vi "GUI_HTT_CTRLv4_2013.vi"() -> ()   [LabVIEW 2020]
uses:
  Shared/GUI_Template/GUI_master/tcp_new_data_event.ctl
  Shared/GUI_Template/GUI_master/tcp new data cluster.ctl
  <vilib>/Utility/config.llb/Write Key (I32).vi
  <vilib>/Platform/browser.llb/Open URL in Default Browser (string).vi
  <vilib>/Utility/config.llb/NI_LVConfig.lvlib
panel:
  in  "Create Log":bool caption="LogTable"
  in  "Scan":T1(ring)
  out "standard output":string
  in  "LogEpilog":bool caption="LogTable"
  in  "New Google\nExpLog for new day?":bool=TRUE
  in  "LogTable":bool
  in  "PicoL2":bool caption="PicoL GUI"
  in  "1Wire B GUI":bool caption="PicoL GUI"
  out "fire::12":string="fire" caption="fire"
  in  "Wavelength.Channel0::14":enum16{"248", "355", "532", "800", "2940"}(ring)=enum."532"
  in  "Wavelength.Channel1::14":enum16{"248", "355", "532", "800", "2940"}(ring)=enum."800"
  in  "Wavelength.Channel0::13":enum16{"532", "800"}(ring)=enum."800"
  in  "EnergyRange.Channel0::14":T2(ring)=enum."400mJ"
  in  "EnergyRange.Channel1::14":T2(ring)=enum."400mJ"
  in  "EnergyRange.Channel0::13":T3(ring)=enum."200mJ"
  in  "energy.channel 1::14":dbl caption="Energy Gaia" min=0.0 max=200.0 format="%#_13g"
  out "Energy (J)":dbl
  in  "Multiplicator":dbl=15.3
  in  "GUIdevice 14":string="HTT-Energy-S-G"
  in  "Multiplicator":dbl=66.6
  in  "Multiplicator Scatter":dbl=100.0
  out "Energy Scatter (J)":dbl
  out "Energy (J)":dbl
  in  "energy.channel 0::13":dbl caption="Energy Drive" min=0.0 max=10.0 format="%#_13g"
  in  "energy.channel 0::14":dbl caption="Energy Scatter" min=0.0 max=20.0 format="%#_13g"
  in  "GUIdevice 13":string="HTT-Energy-D"
  in  "IR Pt Exp And Comp":bool caption="PicoL GUI"
  in  "Position.Axis 2::10":dbl caption="y/vert." min=-6000.0 max=6000.0
  in  "Position.Axis 3::10":dbl caption="Scatter Mode z" min=-20.0 max=20.0
  in  "Position.Axis 1::10":dbl caption="x/hor." min=-150.0 max=150.0
  in  "Position.Axis 2::11":dbl caption="Translation" min=-50.0 max=50.0
  in  "Position.Axis 3::11":dbl caption="Rotation G1" min=-360.0 max=360.0
  in  "Position.Axis 1::11":dbl caption="Rotation G2" min=-360.0 max=360.0
  in  "Ethernet Powerstrip":bool caption="Google Drive"
  in  "Position.Axis 3::4":dbl caption="z" min=-10.0 max=26.0
  in  "Position.Axis 2::6":dbl caption="Delay Stage" min=-6000.0 max=6000.0
  in  "FilterWheelB1":bool caption="PicoB GUI"
  in  "Search Log":bool caption="PicoL GUI"
  in  "Experiment \n(if, shadow, topjet)":bool caption="PicoL GUI"
  in  "RemoteDesktop":bool caption="PicoL GUI"
  in  "Experiment \n(e-profile, xrays)":bool caption="PicoL GUI"
  in  "IR TC Pointing (17s)":bool caption="PicoL GUI"
  in  "Scatter Depletion":bool caption="PicoL GUI"
  in  "Scatter IR Amps":bool caption="PicoL GUI"
  in  "Drive TC Pt":bool caption="PicoL GUI"
  in  "Gaia Profiles":bool caption="PicoL GUI"
  in  "Gaia Pointing":bool caption="PicoL GUI"
  in  "IR Exp and Comp":bool caption="PicoL GUI"
  in  "HTT Interactive":bool caption="PicoL GUI"
  in  "GUIdevice 12":string="HTT_DG645"
  in  "Delay.Ch C::12":dbl caption="Delay" min=-0.1 max=2.0 format="%#_6e"
  in  "Delay.Ch D::12":dbl caption="Width" min=-0.1 max=2.0 format="%#_6e"
  in  "Amplitude.Ch CD::12":dbl caption="DG645" min=0.5 max=5.0
  in  "Field::1":dbl caption="B-Field" min=0.0 max=10000.0
  in  "Delay.Ch 1::8":dbl caption="Delay" min=0.0 max=10.0 format="%#_6e"
  in  "Width.Ch 1::8":dbl caption="Width" min=0.0 max=1.0 format="%#_6e"
  in  "Amplitude.Ch 1::8":dbl caption="Cam Trig Amp" min=0.0 max=12.0
  in  "1Wire L GUI":bool caption="PicoL GUI"
  in  "Opt. Spectrometer":bool caption="PicoL GUI"
  in  "SingleCamGUI":bool caption="PicoL GUI"
  in  "Exp Editor":bool caption="PicoL GUI"
  in  "DB Editor":bool caption="PicoL GUI"
  in  "AddColumns":bool caption="PicoL GUI"
  in  "GEECSplot":bool caption="PicoL GUI"
  in  "LVStarter":bool caption="PicoL GUI"
  in  "MasterControl":bool caption="PicoL GUI"
  in  "MagSpecGUI":bool caption="PicoL GUI"
  in  "Google Drive":bool
  in  "Depletion Cams":bool caption="PicoL GUI"
  in  "D-L-Cams":bool caption="PicoL GUI"
  in  "Position.Axis 2::5":dbl caption="Mode Out z" min=-150.0 max=150.0
  in  "Position.Axis 1::4":dbl caption="Blade" min=-20.0 max=20.0
  in  "Amplitude.Ch 5::8":dbl caption="Trigger Amplitude (V)" min=0.0 max=12.0
  in  "Position.Axis 3::5":dbl caption="Drive Mode In z" min=-200.0 max=200.0
  in  "Position.Axis 1::5":dbl caption="Mode Out Wedge" min=-150.0 max=150.0
  out "Position.Axis3::2":dbl caption="Rotation G1" min=-180.0 max=180.0 format="%#_13g"
  out "Position.Axis2::2":dbl caption="Rotation G2" min=-180.0 max=180.0 format="%#_13g"
  in  "Position.Axis1::2":dbl caption="Translation" min=-60000.0 max=60000.0 format="%#_13g"
  in  "PicoL":bool caption="PicoL GUI"
  in  "PicoB":bool caption="PicoB GUI"
  in  "AnalogOutput.Channel 0::9":dbl caption="Pressure Ctrl (V)" min=0.0 max=10.0
  in  "Width.Ch 5::8":dbl caption="Opening time (s)" min=0.0 max=0.025 format="%#_6e"
  in  "Jet enable":bool caption="Jet Enable"
  in  "Jet trigger":bool caption="Jet Trigger"
  in  "Position.Axis 3::3":dbl caption="Jet Z" min=-25.0 max=25.0
  in  "Position.Axis 2::3":dbl caption="Jet Y" min=-25.0 max=25.0
  in  "Position.Axis 1::3":dbl caption="Jet X" min=-25.0 max=25.0
  in  "Position.Axis 3::6":dbl caption="Probe delay" min=-100.0 max=100.0
  in  "GUIdevice 11":string="HTT-ESP05"
  in  "GUIdevice 8":string="HTT-BNC"
  in  "GUIdevice 6":string="HTT-ESP04"
  in  "GUIdevice 5":string="HTT-ESP03"
  out "error IO 2":errorcluster
  out "fire::10":string
  out "tcp data event":T4
  in  "UDP error message":string
  in  "GUIdevice 7":string="HTT-Pulsar"
  in  "GUIdevice 2":string="Aerotech-HTT"
  in  "GUIdevice 10":string="HTT-ESP06"
  in  "GUIdevice 4":string="HTT-ESP02"
  in  "GUIdevice 1":string="HTT-MagTeslameter-DTM141"
  in  "GUIdevice 3":string="HTT-ESP01"
  in  "GUIdevice 9":string="HTT-HighPressureDAQ"
  in  "Delay.Ch 5::8":dbl caption="Jet timing (s)" min=0.0 max=10.0 format="%#_6e"
  in  "stop":bool
  # "Energy"
  # "CAP"
  # "HTT CONTROL CENTER"
  # "v0.5   04/01/2020"
  # "Drive"
  # "Gas Jet"
  # "GUI Collection"
  # "Compressor"
  # "Drive Cameras"
  # "Mode Imager"
  # "Probe Delay Line"
  # "Scatter Cameras"
  # "Scatter"
  # "Compressor"
  # "Electronics"
  # "BNC"
  # "Mode Imager"
  # "Experiment GUIs"
  # "Scatter Delay vs. Drive"
  # "Turning Mirror"
  # "MC Links"
  # "Docu"
  # "Log Maker"
  # "Energy"
  # "Drive"
  # "Scatter"
  # "Gaia"
  # "Adjustment GUIs"
  # "Range"
  # "Wavelength"
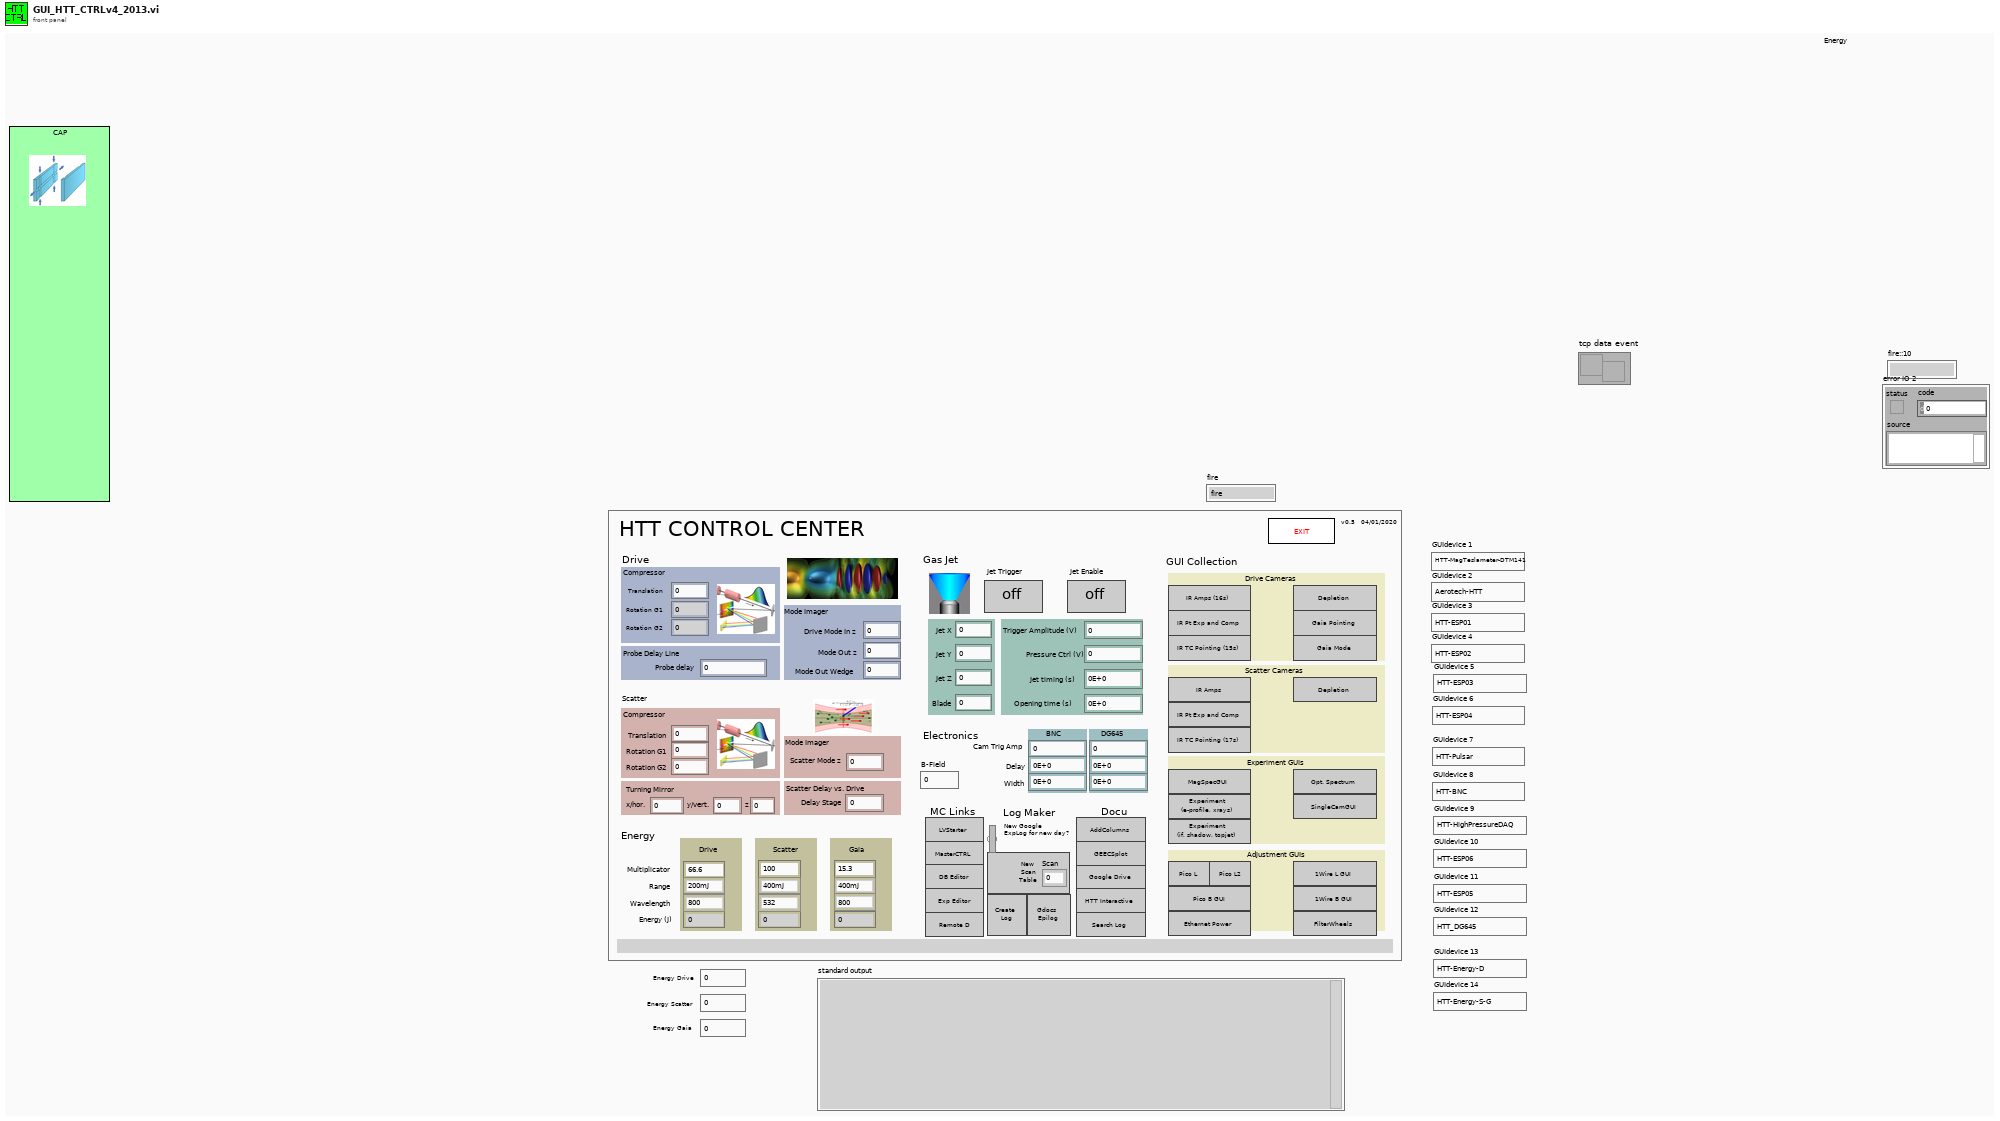
[diagram p1: front panel]
types:
  T1 = enum16{"0", "1", "2", "3", "4", "5", "6", "7", "8", "9", "10", "11", "12", "13", "14", "15", "16", "17", "18", "19", "20", "21", "22", "23", "24", "25", "26", "27", "28", "29", "30", "31", "32", "33", "34", "35", "36", "37", "38", "39", "40", "41", "42", "43", "44", "45", "46", "47", "48", "49", "50", "51", "52", "53", "54", "55", "56", "57", "58", "59", "60", "61", "62", "63", "64", "65", "66", "67", "68", "69", "70", "71", "72", "73", "74", "75", "76", "77", "78", "79", "81", "82", "83", "84", "85", "86", "87", "88", "89", "90", "91", "92", "93", "94", "95", "96", "97", "98", "99", ""}
  T2 = enum16{"4.00mJ", "40.0mJ", "400mJ", "4.00J", "20.00J"}
  T3 = enum16{"2.00mJ", "20.0mJ", "200mJ", "2.00J", "10J"}
  T4 = typedef "tcp_new_data_event.ctl" = refnum<user-event>
  T5 = typedef "tcp new data cluster.ctl" = cluster{"EventEnum":enum16{"new data", "connection status update"}, "Device name":string}
  T6 = enum32{"invalid app kind", "Development System", "Run Time System", "Student Edition", "Embedded LabVIEW", "Evaluation", "Custom"}
  T7 = enum32{"Invalid", "Standard", "Closed", "Hidden", "Minimized", "Maximized"}
  T8 = cluster{"Core":cluster{"Current VI Reference":refnum<vi>, "Close Panel on Exit?":bool}, "Heater timing offset":dbl, "Discharge timing offset":dbl, "Jet trigger":bool, "Tik1":u32, "Tik2":u32, "Fire Continues Allowed":bool, "Jet enable":bool}
  T9 = typedef "imagedata.ctl" = cluster{"image type":i32, "image depth":i32, "image":u8[], "mask":u8[], "colors":u32[], "Rectangle":cluster{"left":i16, "top":i16, "right":i16, "bottom":i16}}
  T10 = typedef "NI_LVConfig.lvlib/Config Data RefNum.ctl" = refnum<k1>
  T11 = cluster{"Current VI Reference":refnum<vi>, "Close Panel on Exit?":bool}
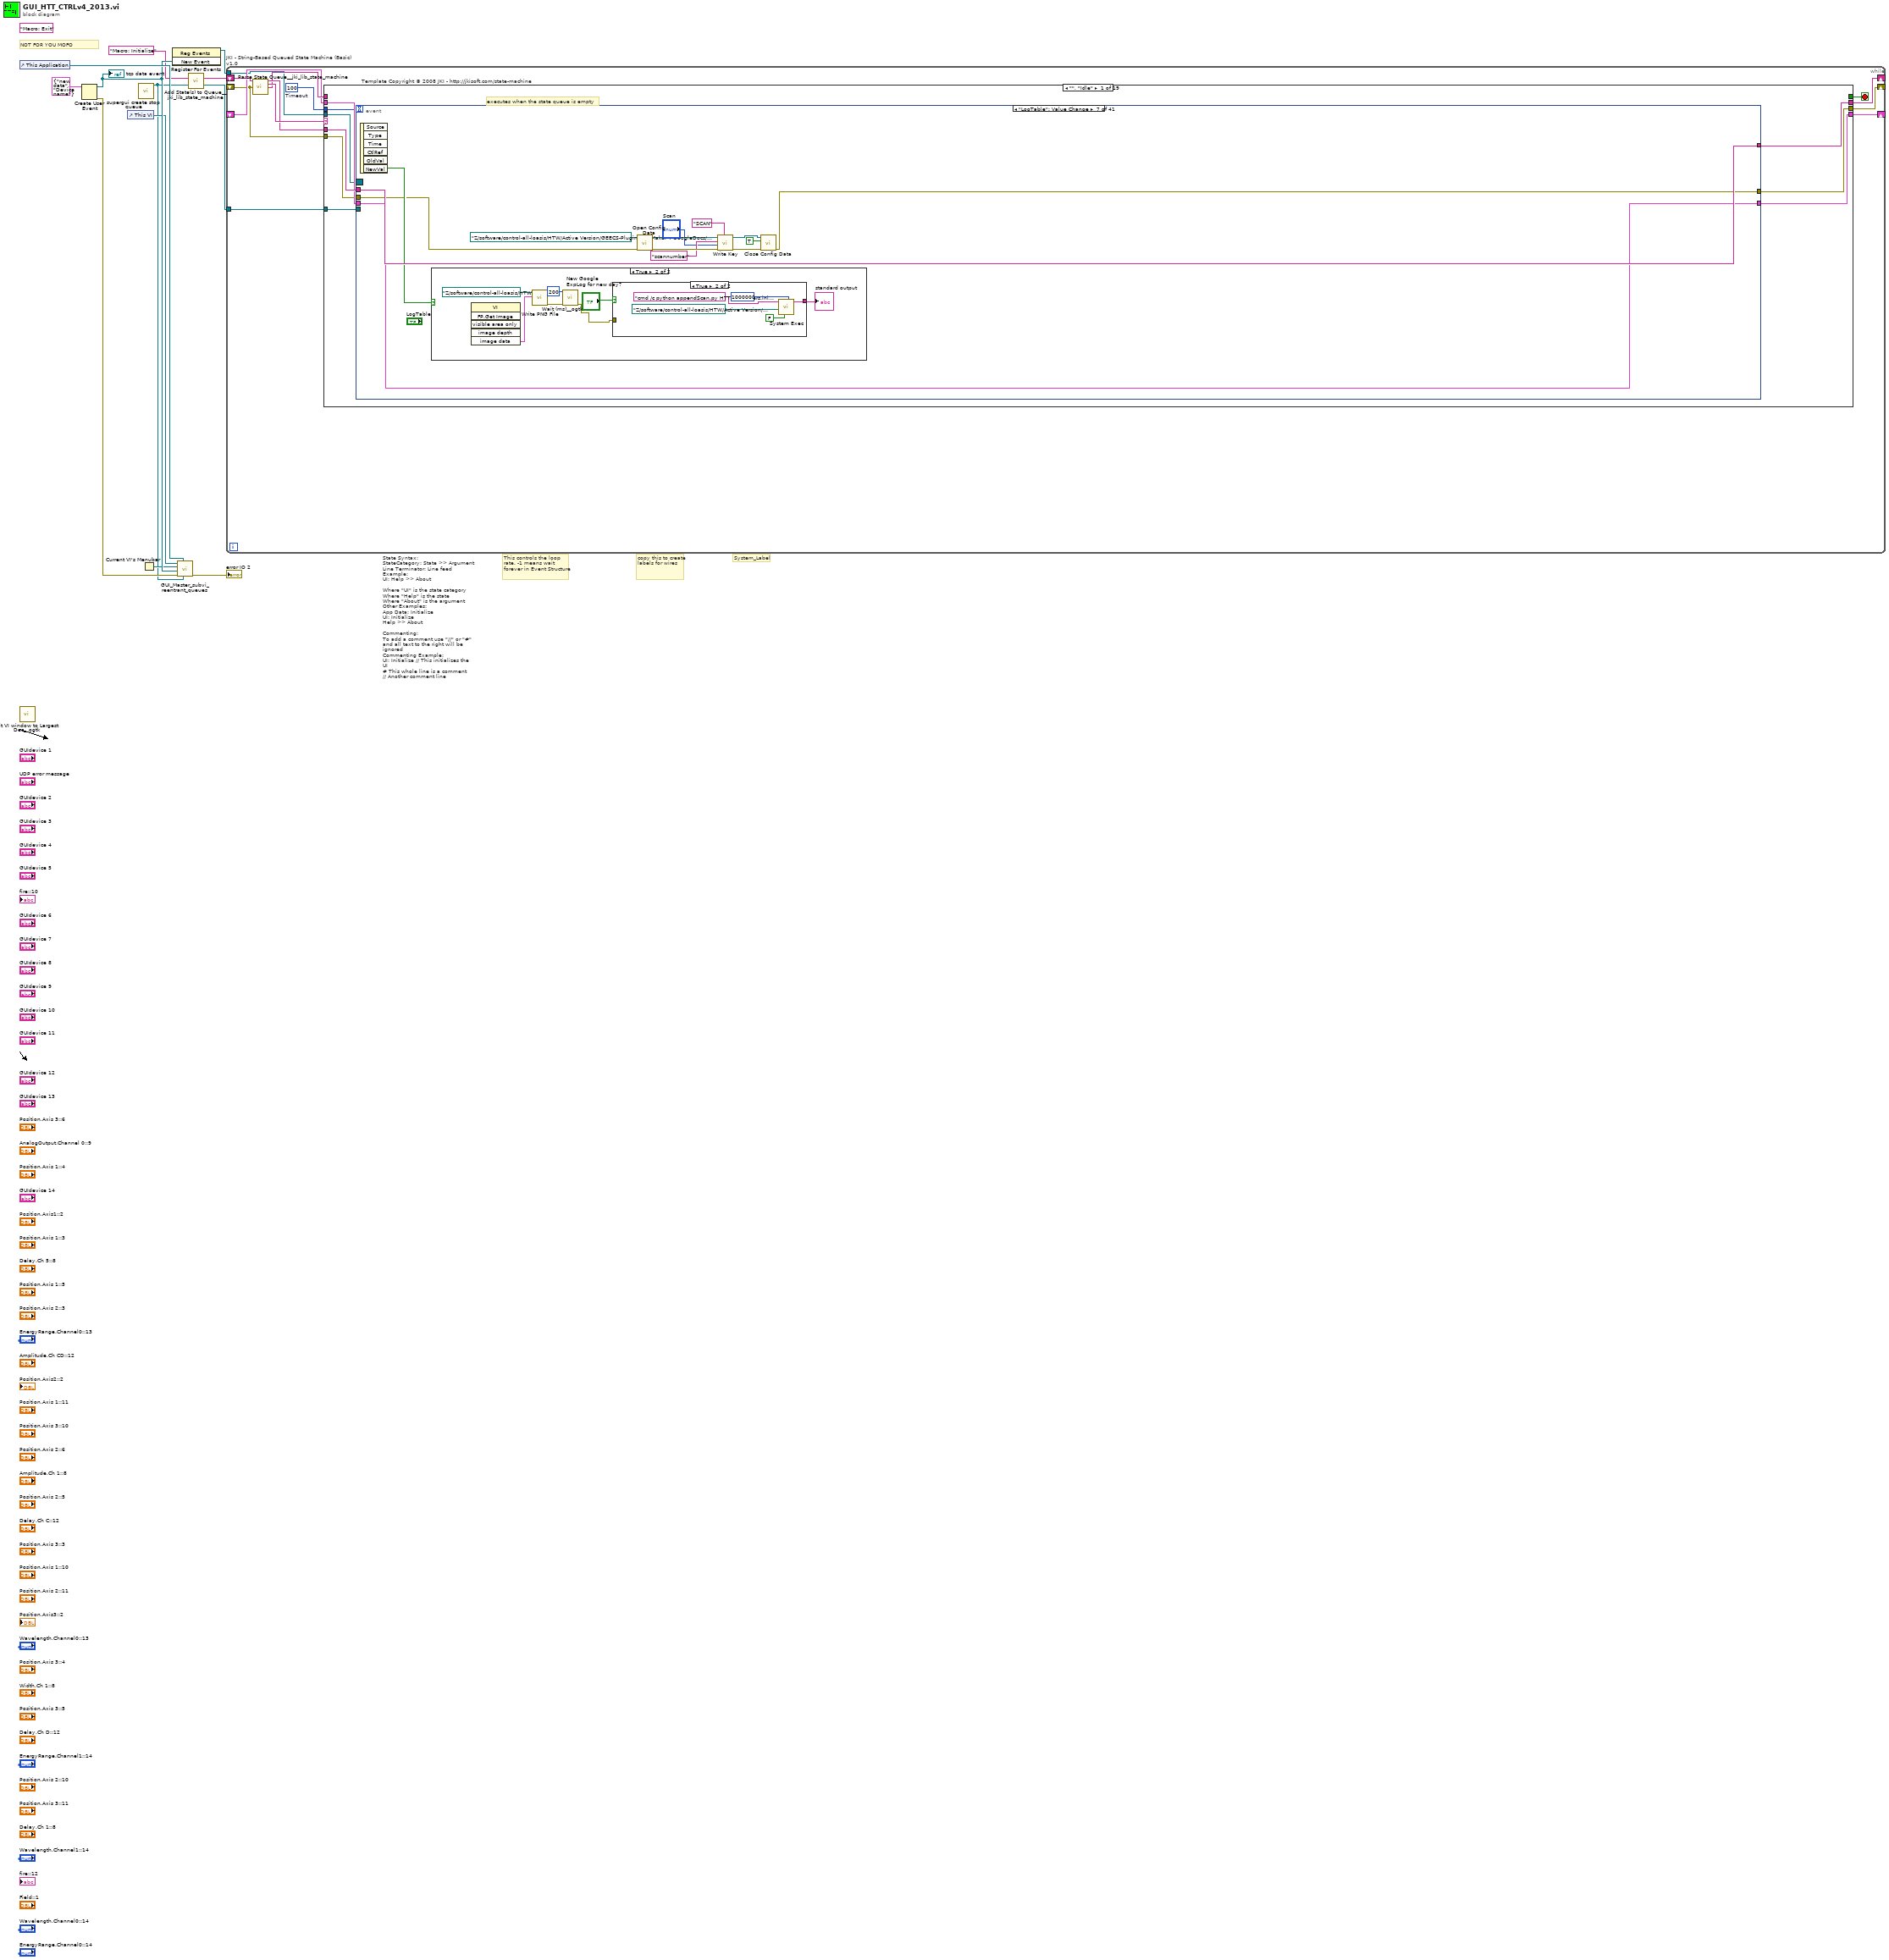
[diagram p0: block diagram]
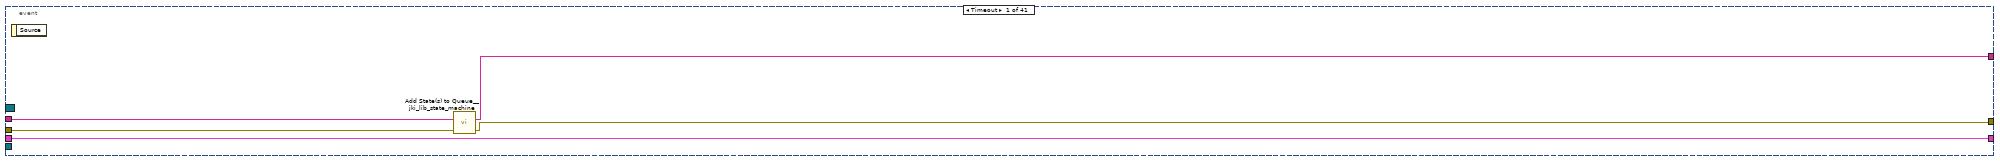
[diagram p2: hidden frame]
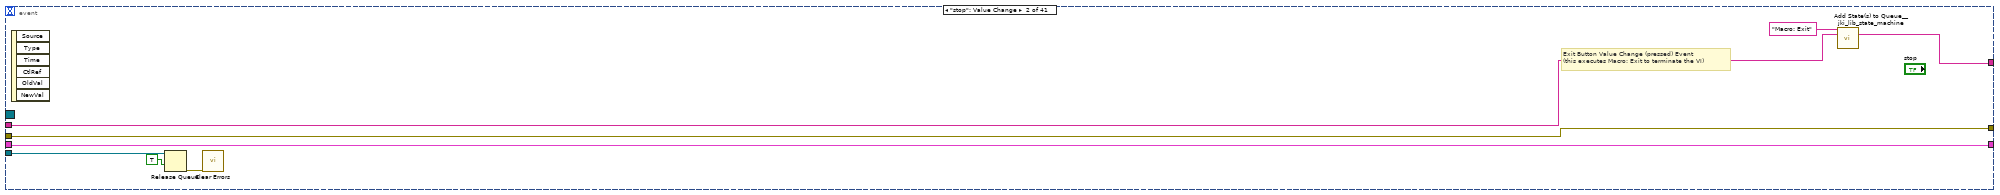
[diagram p3: hidden frame]
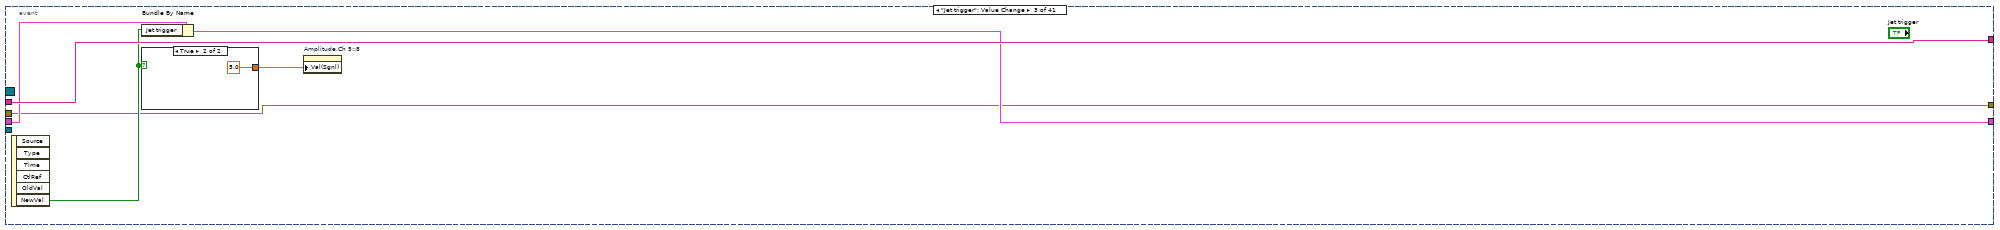
[diagram p4: hidden frame]
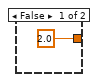
[diagram p5: hidden frame]
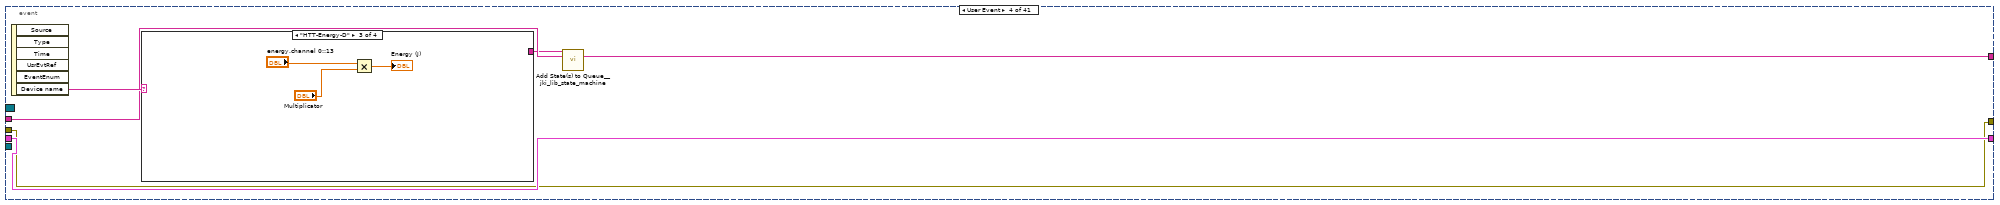
[diagram p6: hidden frame]
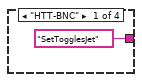
[diagram p7: hidden frame]
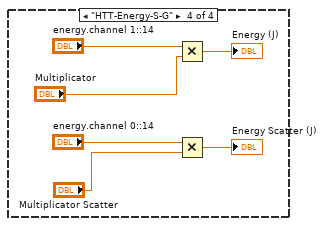
[diagram p9: hidden frame]
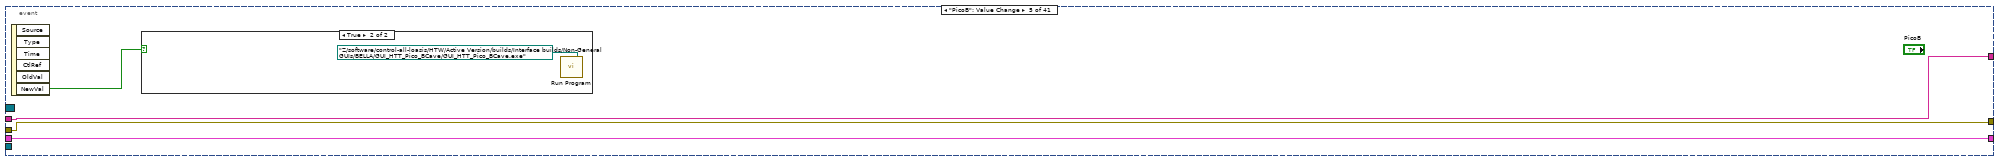
[diagram p10: hidden frame]
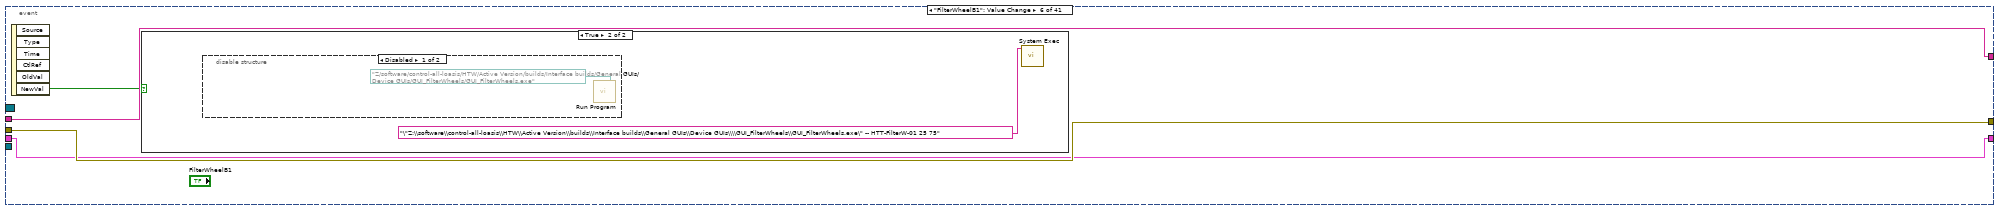
[diagram p12: hidden frame]
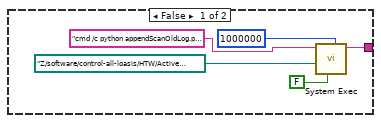
[diagram p16: hidden frame]
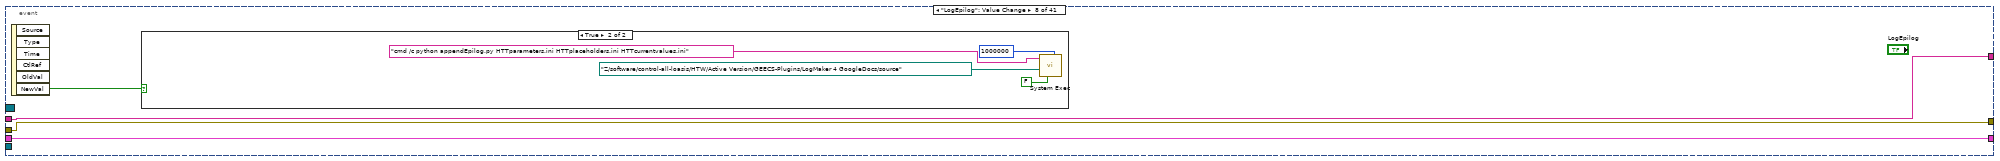
[diagram p17: hidden frame]
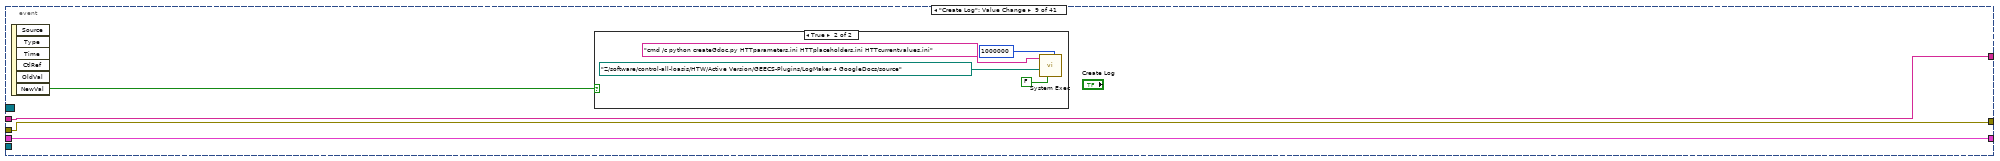
[diagram p19: hidden frame]
diagram:
  (unwired) "Macro: Exit"
  # "State Syntax:\nStateCategory: State >> Argument\nLine Terminator: Line feed\nExample:\nUI: Help >> About\n\nWhere \"UI\" is the state category\nWhere \"Help\" is the state\nWhere \"About\" is the argument\nOther Examples:\nApp Data: Initialize\nUI: Initialize\nHelp >> About\n\nCommenting:\nTo add a comment use \"//\" or \"#\" and all text to the right will be ignored\nCommenting Example:\nUI: Initialize // This initializes the UI\n# This whole line is a comment\n// Another comment line"
  # "copy this to create labels for wires"
  # "This controls the loop rate. -1 means wait forever in Event Structure"
  # "System_Label"
  # "NOT FOR YOU MOFO"
  n1 = control-ref of="This Application"() -> (w11:refnum<vi>)
  n2 = call <userlib>:"Fit VI window to Largest Dec__ogtk.vi"() -> ()  [unwired: 6 in, 2 out]
  n3 = Create User Event(user event datatype=T5 {"EventEnum"=enum."new data", "Device name"="Device name"} ("New Event")) -> (user event=w10:refnum<user-event>, error out=w9:errorcluster)  [unwired: 1 in]
  "tcp data event" <- w10
  n4 = control-ref of="This VI"() -> (w5:refnum<vi>)
  n5 = call "supergui create stop queue.vi"() -> ("STOP Queue out"=w2:refnum<queue>)  [unwired: 11 in]
  n6 = Current VI's Menubar() -> (w7:refnum<k9>)
  n7 = register-events(w10) -> (reference out=w1:refnum<event-registration>)  [unwired: 2 in, 1 out]
  n8 = call "GUI_Master_subvi_reentrant_queues.vi"("STOP Queue in"=w2, "This Application"=w11, "error in (no error)"=w9, "tcp data event"=w10, "Caller menu reference"=w7, "Caller VI ref"=w5) -> ("error out"=→"error IO 2":errorcluster)  [unwired: 5 in]
  n9 = call <vilib>:"Add State(s) to Queue__jki_lib_state_machine.vi"("State(s) in (\"\")"="Macro: Initialize") -> ("States Out"=w3:string)  [unwired: 14 in]
  n10 = while "JKI - String-Based Queued State Machine (Basic) v1.0" {
    shift-right: [w18] -> _
    shift-left: _ -> [w17]
    shift-right: [w20] -> _
    shift-left: _ -> [w15]
    shift-right: [w19] -> _
    shift-left: w3 -> [w21]
    tunnel: w1 -> [w14]
    tunnel: w2 -> [w13]
    stop <- w12 stop-if-true
    w16 = 100  # Timeout
    # "Template Copyright © 2008 JKI - http://jkisoft.com/state-machine"
    n11 = call <vilib>:"Parse State Queue__jki_lib_state_machine.vi"("State Queue"=w21, "Error In (no error)"=w15) -> ("Remaining States"=w23:string, "Current State"=w24:string, "Arguments"=w22:string)  [unwired: 11 in]
    n12 = case shown="\"\", \"Idle\"" w24 {
      selector: w24 -> [_ _ _ w311 _ _ _ _ _ _ _ _ _ _ _ _ _ _ _]
      tunnel: w23 -> [w33 w305 w310 w315 w333 w339 w344 w348 w360 w366 w370 w374 w380 w391 w417 w422 w432 w436 w442]
      tunnel: w22 -> [_ _ _ _ _ _ _ _ _ _ _ _ w375 w385 _ _ _ _ _]
      tunnel: w17 -> [w31 w306 w307 w313 w324 w336 w342 w345 _ w361 w367 w372 w378 w387 w414 w419 w429 w433 w440]
      tunnel: [w30 w304 w308 w317 w330 errorcluster {"status"=FALSE, "code"=0, "source"=""} ("error out") w341 w346 w357 w362 w368 w371 w376 w388 w415 w420 w430 w434 w437] -> w20
      tunnel: w15 -> [w29 w304 w308 w316 w330 w335 w341 w346 w357 w363 w368 w371 w377 w389 w415 w420 w430 w434 w438]
      tunnel: [w32 w305 w309 w314 w332 w338 w343 w347 w359 w365 w369 w373 w379 w390 w416 w421 w431 w435 w441] -> w19
      tunnel: [_ _ _ _ _ _ TRUE _ _ _ _ _ _ _ _ _ _ _ _] -> w12
      tunnel: [w25 w306 w307 w313 w331 w336 w342 w345 w358 w361 w367 w372 w378 w387 w414 w419 w429 w433 w440] -> w18
      tunnel: w16 -> [w28 _ _ _ _ _ _ _ _ _ _ _ _ _ _ _ _ _ _]
      tunnel: w14 -> [w27 _ _ _ _ _ _ _ _ _ _ _ _ _ _ _ _ _ _]
      tunnel: w13 -> [w26 _ _ _ _ _ _ _ _ _ _ _ _ _ _ _ _ _ _]
      frame "", "Idle" {
        # "executes when the state queue is empty"
        n13 = event shown="[6] \"LogTable\": Value Change" {
          selector: w27 -> [_ _ _ _ _ _ _ _ _ _ _ _ _ _ _ _ _ _ _ _ _ _ _ _ _ _ _ _ _ _ _ _ _ _ _ _ _ _ _ _ _]
          dyn-events: _ -> [_ _ _ _ _ _ _ _ _ _ _ _ _ _ _ _ _ _ _ _ _ _ _ _ _ _ _ _ _ _ _ _ _ _ _ _ _ _ _ _ _]
          timeout: w28 -> [_ _ _ _ _ _ _ _ _ _ _ _ _ _ _ _ _ _ _ _ _ _ _ _ _ _ _ _ _ _ _ _ _ _ _ _ _ _ _ _ _]
          tunnel: w33 -> [w37 w45 w51 w57 w73 w78 w94 w115 w123 w131 w136 w141 w146 w151 w156 w161 w166 w171 w176 w181 w186 w191 w196 w201 w206 w211 w216 w221 w226 w231 w236 w241 w246 w251 w256 w261 w266 w271 w276 w283 w291]
          tunnel: [w36 w44 w51 w56 w73 w78 w94 w115 w123 w131 w136 w141 w146 w151 w156 w161 w166 w171 w176 w181 w186 w191 w196 w201 w206 w211 w216 w221 w226 w231 w236 w241 w246 w251 w256 w261 w266 w271 w276 w283 w290] -> w32
          tunnel: w31 -> [w34 w42 w50 w58 w70 w75 w92 w112 w120 w128 w133 w138 w143 w148 w153 w158 w163 w168 w173 w178 w183 w188 w193 w198 w203 w208 w213 w218 w223 w228 w233 w238 w243 w248 w253 w258 w263 w268 w273 w282 w288]
          tunnel: [w35 w43 w47 w55 w71 w76 w81 w113 w121 w129 w134 w139 w144 w149 w154 w159 w164 w169 w174 w179 w184 w189 w194 w199 w204 w209 w214 w219 w224 w229 w234 w239 w244 w249 w254 w259 w264 w269 w274 w278 w289] -> w30
          tunnel: w29 -> [w35 w43 w47 w55 w71 w76 w82 w113 w121 w129 w134 w139 w144 w149 w154 w159 w164 w169 w174 w179 w184 w189 w194 w199 w204 w209 w214 w219 w224 w229 w234 w239 w244 w249 w254 w259 w264 w269 w274 w278 w289]
          tunnel: [w34 w42 w49 w58 w70 w75 w92 w112 w120 w128 w133 w138 w143 w148 w153 w158 w163 w168 w173 w178 w183 w188 w193 w198 w203 w208 w213 w218 w223 w228 w233 w238 w243 w248 w253 w258 w263 w268 w273 w281 w288] -> w25
          tunnel: w26 -> [_ w39 _ _ _ _ _ _ _ _ _ _ _ _ _ _ _ _ _ _ _ _ _ _ _ _ _ _ _ _ _ _ _ _ _ _ _ _ _ _ _]
          event Timeout {
            n14 = event-data() -> ()  [unwired: 1 in, 1 out]
            n15 = call <vilib>:"Add State(s) to Queue__jki_lib_state_machine.vi"("State(s) in (\"\")"=w37) -> ("States Out"=w36:string)  [unwired: 14 in]
          }
          event "stop": Value Change {
            # "Exit Button Value Change (pressed) Event\n(this executes Macro: Exit to terminate the VI)"
            n16 = event-data() -> ()  [unwired: 1 in, 6 out]
            n17 = Release Queue(queue=w39, force destroy? (F)=TRUE) -> (error out=w40:errorcluster)  [unwired: 1 in, 2 out]
            n18 = call <vilib>:"Clear Errors.vi"("error in (no error)"=w40) -> ()  [unwired: 5 in, 2 out]
            n19 = call <vilib>:"Add State(s) to Queue__jki_lib_state_machine.vi"("State(s) in Front (\"\")"="Macro: Exit", "State(s) in (\"\")"=w45) -> ("States Out"=w44:string)  [unwired: 13 in]
          }
          event "Jet trigger": Value Change {
            n20 = event-data() -> ("NewVal"=w48:bool)  [unwired: 1 in, 5 out]
            n21 = Bundle By Name(cluster=w50, "Jet trigger"=w48) -> (w49:T8)
            n22 = case shown="True" w48 {
              tunnel: [2.0 ("Amplitude.Ch CD::10") 5.0 ("Amplitude.Ch CD::10")] -> w46
              frame False {
              }
              frame True {
              }
            }
            n23 = property on="Amplitude.Ch 5::8" class="DigNum (strict)"("Val(Sgnl)"=w46) -> ()  [unwired: 2 in, 2 out]
          }
          event User Event {
            n24 = event-data() -> ("Device name"=w59:string)  [unwired: 1 in, 5 out]
            n25 = case shown="\"HTT-Energy-D\"" w59 {
              tunnel: ["SetTogglesJet" _ _ _] -> w54
              frame "HTT-BNC" {
              }
              frame "False", Default {
              }
              frame "HTT-Energy-D" {
                n26 = Multiply(x="energy.channel 0::13", y="Multiplicator") -> (x*y=→"Energy (J)":dbl)
              }
              frame "HTT-Energy-S-G" {
                n27 = Multiply(x="energy.channel 1::14", y="Multiplicator") -> (x*y=→"Energy (J)":dbl)
                n28 = Multiply(x="energy.channel 0::14", y="Multiplicator Scatter") -> (x*y=→"Energy Scatter (J)":dbl)
              }
            }
            n29 = call <vilib>:"Add State(s) to Queue__jki_lib_state_machine.vi"("State(s) in Front (\"\")"=w54, "State(s) in (\"\")"=w57) -> ("States Out"=w56:string)  [unwired: 13 in]
          }
          event "PicoB": Value Change {
            n30 = event-data() -> ("NewVal"=w72:bool)  [unwired: 1 in, 5 out]
            n31 = case shown="True" w72 {
              frame False {
              }
              frame True {
                n32 = call "Run Program.vi"("Program Path"=path "Z:/software/control-all-loasis/HTW/Active Version/builds/Interface builds/Non-General GUIs/BELLA/GUI_HTT_Pico_BCave/GUI_HTT_Pico_BCave.exe") -> ()  [unwired: 1 in]
              }
            }
          }
          event "FilterWheelB1": Value Change {
            n33 = event-data() -> ("NewVal"=w77:bool)  [unwired: 1 in, 5 out]
            n34 = case shown="True" w77 {
              frame False {
              }
              frame True {
                n35 = disable-structure shown="Disabled" {
                  frame Disabled {
                    n36 = call "Run Program.vi"("Program Path"=path "Z:/software/control-all-loasis/HTW/Active Version/builds/Interface builds/General GUIs/Device GUIs/GUI_FilterWheels/GUI_FilterWheels.exe") -> ()  [unwired: 1 in]
                  }
                  frame Enabled {
                  }
                }
                n37 = call <vilib>:"System Exec.vi"("command line"="\"Z:\\software\\control-all-loasis\\HTW\\Active Version\\builds\\Interface builds\\General GUIs\\Device GUIs\\\\GUI_FilterWheels\\GUI_FilterWheels.exe\" -- HTT-FilterW-01 25 75") -> ()  [unwired: 7 in, 4 out]
              }
            }
          }
          event "LogTable": Value Change {
            n38 = event-data() -> ("NewVal"=w93:bool)  [unwired: 1 in, 5 out]
            n39 = case shown="True" w93 {
              frame False {
              }
              frame True {
                n40 = invoke class="VI" method="FP.Get Image"() -> ("image data"=w101:T9)  [unwired: 6 in, 5 out]
                n41 = call <vilib>:"Write PNG File.vi"("image data"=w101, "path to PNG file"=path "Z:/software/control-all-loasis/HTW/Active Version/GEECS-Plugins/LogMaker 4 GoogleDocs/source/frontpanel.png" ("report file path")) -> ("error out"=w96:errorcluster)  [unwired: 8 in, 1 out]
                n42 = call <userlib>:"Wait (ms)__ogtk.vi"("error in (no error)"=w96, "milliseconds to wait"=u32 200 ("millisecond timer value")) -> ("error out"=w95:errorcluster)  [unwired: 8 in, 1 out]
                n43 = case shown="True" "New Google\nExpLog for new day?" {
                  tunnel: [w102 w107] -> w98
                  tunnel: w95 -> [_ _]
                  frame False {
                    n44 = call <vilib>:"System Exec.vi"("expected output size  (4096)"=u32 1000000, "run minimized? (F)"=FALSE, "working directory"=path "Z:/software/control-all-loasis/HTW/Active Version/GEECS-Plugins/LogMaker 4 GoogleDocs/source", "command line"="cmd /c python appendScanOldLog.py HTTparameters.ini HTTplaceholders.ini HTTcurrentvalues.ini") -> ("standard output"=w102:string)  [unwired: 4 in, 3 out]
                  }
                  frame True {
                    n45 = call <vilib>:"System Exec.vi"("expected output size  (4096)"=u32 1000000, "run minimized? (F)"=FALSE, "working directory"=path "Z:/software/control-all-loasis/HTW/Active Version/GEECS-Plugins/LogMaker 4 GoogleDocs/source", "command line"="cmd /c python appendScan.py HTTparameters.ini HTTplaceholders.ini HTTcurrentvalues.ini") -> ("standard output"=w107:string)  [unwired: 4 in, 3 out]
                  }
                }
                "standard output" <- w98
              }
            }
            n46 = call <vilib>:"Open Config Data.vi"("error in (no error)"=w82, "configuration file path"=path "Z:/software/control-all-loasis/HTW/Active Version/GEECS-Plugins/LogMaker 4 GoogleDocs/source/HTTparameters.ini") -> ("error out"=w88:errorcluster, "refnum"=w90:T10)  [unwired: 7 in, 1 out]
            n47 = call-poly <vilib>:"Write Key.vi"("section"="SCAN", "error in (no error)"=w88, "value"="Scan", "key"="scannumber", "refnum"=w90) -> ("error out"=w87:errorcluster, "refnum out"=w89:T10)  [unwired: 4 in, 1 out]
            n48 = call <vilib>:"Close Config Data.vi"("error in (no error)"=w87, "write file if changed (T)"=TRUE, "refnum"=w89) -> ("error out"=w81:errorcluster)  [unwired: 7 in, 1 out]
          }
          event "LogEpilog": Value Change {
            n49 = event-data() -> ("NewVal"=w114:bool)  [unwired: 1 in, 5 out]
            n50 = case shown="True" w114 {
              frame False {
              }
              frame True {
                n51 = call <vilib>:"System Exec.vi"("expected output size  (4096)"=u32 1000000, "run minimized? (F)"=FALSE, "working directory"=path "Z:/software/control-all-loasis/HTW/Active Version/GEECS-Plugins/LogMaker 4 GoogleDocs/source", "command line"="cmd /c python appendEpilog.py HTTparameters.ini HTTplaceholders.ini HTTcurrentvalues.ini") -> ()  [unwired: 4 in, 4 out]
              }
            }
          }
          event "Create Log": Value Change {
            n52 = event-data() -> ("NewVal"=w122:bool)  [unwired: 1 in, 5 out]
            n53 = case shown="True" w122 {
              frame False {
              }
              frame True {
                n54 = call <vilib>:"System Exec.vi"("expected output size  (4096)"=u32 1000000, "run minimized? (F)"=FALSE, "working directory"=path "Z:/software/control-all-loasis/HTW/Active Version/GEECS-Plugins/LogMaker 4 GoogleDocs/source", "command line"="cmd /c python createGdoc.py HTTparameters.ini HTTplaceholders.ini HTTcurrentvalues.ini") -> ()  [unwired: 4 in, 4 out]
              }
            }
          }
          event "PicoL": Value Change {
            n55 = event-data() -> ("NewVal"=w130:bool)  [unwired: 1 in, 5 out]
            n56 = case shown="True" w130 {
              frame False {
              }
              frame True {
                n57 = call "Run Program.vi"("Program Path"=path "Z:/software/control-all-loasis/HTW/Active Version/builds/Interface builds/Non-General GUIs/BELLA/GUI_HTT_Pico_LCave/GUI_HTT_Pico_LCave.exe") -> ()  [unwired: 1 in]
              }
            }
          }
          event "PicoL2": Value Change {
            n58 = event-data() -> ("NewVal"=w135:bool)  [unwired: 1 in, 5 out]
            n59 = case shown="True" w135 {
              frame False {
              }
              frame True {
                n60 = call "Run Program.vi"("Program Path"=path "Z:/software/control-all-loasis/HTW/Active Version/builds/Interface builds/Non-General GUIs/BELLA/GUI_HTT_Pico_LCave2/GUI_HTT_Pico_LCave2.exe") -> ()  [unwired: 1 in]
              }
            }
          }
          event "D-L-Cams": Value Change {
            n61 = event-data() -> ("NewVal"=w140:bool)  [unwired: 1 in, 5 out]
            n62 = case shown="True" w140 {
              frame False {
              }
              frame True {
                n63 = call "Run Program.vi"("Program Path"=path "Z:/software/control-all-loasis/HTW/Active Version/builds/Interface builds/Non-General GUIs/BELLA/GUI_HTT_MultiCam/GUI_HTT_MultiCamsDriveAmp.exe") -> ()  [unwired: 1 in]
              }
            }
          }
          event "Depletion Cams": Value Change {
            n64 = event-data() -> ("NewVal"=w145:bool)  [unwired: 1 in, 5 out]
            n65 = case shown="True" w145 {
              frame False {
              }
              frame True {
                n66 = call "Run Program.vi"("Program Path"=path "Z:/software/control-all-loasis/HTW/Active Version/builds/Interface builds/Non-General GUIs/BELLA/GUI_HTT_MultiCam/GUI_HTT_MultiCamsDriveDepletion.exe") -> ()  [unwired: 1 in]
              }
            }
          }
          event "Gaia Profiles": Value Change {
            n67 = event-data() -> ("NewVal"=w150:bool)  [unwired: 1 in, 5 out]
            n68 = case shown="True" w150 {
              frame False {
              }
              frame True {
                n69 = call "Run Program.vi"("Program Path"=path "Z:/software/control-all-loasis/HTW/Active Version/builds/Interface builds/Non-General GUIs/BELLA/GUI_HTT_MultiCam/GUI_HTT_MultiCamsDriveGaiaProfile.exe") -> ()  [unwired: 1 in]
              }
            }
          }
          event "Drive TC Pt": Value Change {
            n70 = event-data() -> ("NewVal"=w155:bool)  [unwired: 1 in, 5 out]
            n71 = case shown="True" w155 {
              frame False {
              }
              frame True {
                n72 = call "Run Program.vi"("Program Path"=path "Z:/software/control-all-loasis/HTW/Active Version/builds/Interface builds/Non-General GUIs/BELLA/GUI_HTT_MultiCam/GUI_HTT_MultiCamsDriveTCPointing.exe") -> ()  [unwired: 1 in]
              }
            }
          }
          event "Scatter IR Amps": Value Change {
            n73 = event-data() -> ("NewVal"=w160:bool)  [unwired: 1 in, 5 out]
            n74 = case shown="True" w160 {
              frame False {
              }
              frame True {
                n75 = call "Run Program.vi"("Program Path"=path "Z:/software/control-all-loasis/HTW/Active Version/builds/Interface builds/Non-General GUIs/BELLA/GUI_HTT_MultiCam/GUI_HTT_MultiCamsScatterAmp.exe") -> ()  [unwired: 1 in]
              }
            }
          }
          event "Scatter Depletion": Value Change {
            n76 = event-data() -> ("NewVal"=w165:bool)  [unwired: 1 in, 5 out]
            n77 = case shown="True" w165 {
              frame False {
              }
              frame True {
                n78 = call "Run Program.vi"("Program Path"=path "Z:/software/control-all-loasis/HTW/Active Version/builds/Interface builds/Non-General GUIs/BELLA/GUI_HTT_MultiCam/GUI_HTT_MultiCamsScatterDepletion.exe") -> ()  [unwired: 1 in]
              }
            }
          }
          event "IR Exp and Comp": Value Change {
            n79 = event-data() -> ("NewVal"=w170:bool)  [unwired: 1 in, 5 out]
            n80 = case shown="True" w170 {
              frame False {
              }
              frame True {
                n81 = call "Run Program.vi"("Program Path"=path "Z:/software/control-all-loasis/HTW/Active Version/builds/Interface builds/Non-General GUIs/BELLA/GUI_HTT_MultiCam/GUI_HTT_MultiCamsDriveExpAndComp.exe") -> ()  [unwired: 1 in]
              }
            }
          }
          event "Gaia Pointing": Value Change {
            n82 = event-data() -> ("NewVal"=w175:bool)  [unwired: 1 in, 5 out]
            n83 = case shown="True" w175 {
              frame False {
              }
              frame True {
                n84 = call "Run Program.vi"("Program Path"=path "Z:/software/control-all-loasis/HTW/Active Version/builds/Interface builds/Non-General GUIs/BELLA/GUI_HTT_MultiCam/GUI_HTT_MultiCamsDriveGaiaPointing.exe") -> ()  [unwired: 1 in]
              }
            }
          }
          event "1Wire L GUI": Value Change {
            n85 = event-data() -> ("NewVal"=w180:bool)  [unwired: 1 in, 5 out]
            n86 = case shown="True" w180 {
              frame False {
              }
              frame True {
                n87 = call "Run Program.vi"("Program Path"=path "Z:/software/control-all-loasis/HTW/Active Version/builds/Interface builds/Non-General GUIs/BELLA/GUI_HTT_1Wire/GUI_HTT_1Wire.exe") -> ()  [unwired: 1 in]
              }
            }
          }
          event "1Wire B GUI": Value Change {
            n88 = event-data() -> ("NewVal"=w185:bool)  [unwired: 1 in, 5 out]
            n89 = case shown="True" w185 {
              frame False {
              }
              frame True {
                n90 = call "Run Program.vi"("Program Path"=path "Z:/software/control-all-loasis/HTW/Active Version/builds/Interface builds/Non-General GUIs/BELLA/GUI_HTT_1Wire_BCave/GUI_HTT_1Wire_BCave.exe") -> ()  [unwired: 1 in]
              }
            }
          }
          event "MagSpecGUI": Value Change {
            n91 = event-data() -> ("NewVal"=w190:bool)  [unwired: 1 in, 5 out]
            n92 = case shown="True" w190 {
              frame False {
              }
              frame True {
                n93 = call "Run Program.vi"("Program Path"=path "Z:/software/control-all-loasis/HTW/Active Version/builds/Interface builds/Non-General GUIs/BELLA/GUI_HTT_MultiCam/GUI_HTT_MultiCamsDriveMagSpec.exe") -> ()  [unwired: 1 in]
              }
            }
          }
          event "IR TC Pointing (17s)": Value Change {
            n94 = event-data() -> ("NewVal"=w195:bool)  [unwired: 1 in, 5 out]
            n95 = case shown="True" w195 {
              frame False {
              }
              frame True {
                n96 = call "Run Program.vi"("Program Path"=path "Z:/software/control-all-loasis/HTW/Active Version/builds/Interface builds/Non-General GUIs/BELLA/GUI_HTT_MultiCam/GUI_HTT_MultiCamsScatterTCPointing.exe") -> ()  [unwired: 1 in]
              }
            }
          }
          event "IR Pt Exp And Comp": Value Change {
            n97 = event-data() -> ("NewVal"=w200:bool)  [unwired: 1 in, 5 out]
            n98 = case shown="True" w200 {
              frame False {
              }
              frame True {
                n99 = call "Run Program.vi"("Program Path"=path "Z:/software/control-all-loasis/HTW/Active Version/builds/Interface builds/Non-General GUIs/BELLA/GUI_HTT_MultiCam/GUI_HTT_MultiCamsScatterExpAndComp.exe") -> ()  [unwired: 1 in]
              }
            }
          }
          event "Experiment \n(e-profile, xrays)": Value Change {
            n100 = event-data() -> ("NewVal"=w205:bool)  [unwired: 1 in, 5 out]
            n101 = case shown="True" w205 {
              frame False {
              }
              frame True {
                n102 = call "Run Program.vi"("Program Path"=path "Z:/software/control-all-loasis/HTW/Active Version/builds/Interface builds/Non-General GUIs/BELLA/GUI_HTT_MultiCam/GUI_HTT_MultiCamsDriveExperiment1.exe") -> ()  [unwired: 1 in]
              }
            }
          }
          event "Experiment \n(if, shadow, topjet)": Value Change {
            n103 = event-data() -> ("NewVal"=w210:bool)  [unwired: 1 in, 5 out]
            n104 = case shown="True" w210 {
              frame False {
              }
              frame True {
                n105 = call "Run Program.vi"("Program Path"=path "Z:/software/control-all-loasis/HTW/Active Version/builds/Interface builds/Non-General GUIs/BELLA/GUI_HTT_MultiCam/GUI_HTT_MultiCamsDriveExperiment2.exe") -> ()  [unwired: 1 in]
              }
            }
          }
          event "MasterControl": Value Change {
            n106 = event-data() -> ("NewVal"=w215:bool)  [unwired: 1 in, 5 out]
            n107 = case shown="True" w215 {
              frame False {
              }
              frame True {
                n108 = call "Run Program.vi"("Program Path"=path "Z:/software/control-all-loasis/HTW/Active Version/builds/Interface builds/General GUIs/MC/Master Control/Master Control.exe") -> ()  [unwired: 1 in]
              }
            }
          }
          event "LVStarter": Value Change {
            n109 = event-data() -> ("NewVal"=w220:bool)  [unwired: 1 in, 5 out]
            n110 = case shown="True" w220 {
              frame False {
              }
              frame True {
                n111 = call "Run Program.vi"("Program Path"=path "Z:/software/control-all-loasis/HTW/Active Version/builds/Interface builds/General GUIs/MC/LVstarter/LVstarter.exe") -> ()  [unwired: 1 in]
              }
            }
          }
          event "GEECSplot": Value Change {
            n112 = event-data() -> ("NewVal"=w225:bool)  [unwired: 1 in, 5 out]
            n113 = case shown="True" w225 {
              frame False {
              }
              frame True {
                n114 = call "Run Program.vi"("Program Path"=path "P:/10_Software/ajg builds/GEECSplotter 20200129/GEECSplotter.exe") -> ()  [unwired: 1 in]
              }
            }
          }
          event "AddColumns": Value Change {
            n115 = event-data() -> ("NewVal"=w230:bool)  [unwired: 1 in, 5 out]
            n116 = case shown="True" w230 {
              frame False {
              }
              frame True {
                n117 = call "Run Program.vi"("Program Path"=path "P:/10_Software/ajg builds/Add columns to Masterlog 20200213/Add columns to Masterlog.exe") -> ()  [unwired: 1 in]
              }
            }
          }
          event "DB Editor": Value Change {
            n118 = event-data() -> ("NewVal"=w235:bool)  [unwired: 1 in, 5 out]
            n119 = case shown="True" w235 {
              frame False {
              }
              frame True {
                n120 = call "Run Program.vi"("Program Path"=path "Z:/software/control-all-loasis/HTW/Active Version/builds/Interface builds/General GUIs/Database editor/Database editor.exe") -> ()  [unwired: 1 in]
              }
            }
          }
          event "Exp Editor": Value Change {
            n121 = event-data() -> ("NewVal"=w240:bool)  [unwired: 1 in, 5 out]
            n122 = case shown="True" w240 {
              frame False {
              }
              frame True {
                n123 = call "Run Program.vi"("Program Path"=path "Z:/software/control-all-loasis/HTW/Active Version/builds/Interface builds/General GUIs/Database editor/Expt_Devices_GUI_Datagridview.exe") -> ()  [unwired: 1 in]
              }
            }
          }
          event "SingleCamGUI": Value Change {
            n124 = event-data() -> ("NewVal"=w245:bool)  [unwired: 1 in, 5 out]
            n125 = case shown="True" w245 {
              frame False {
              }
              frame True {
                n126 = call "Run Program.vi"("Program Path"=path "Z:/software/control-all-loasis/HTW/Active Version/builds/Interface builds/General GUIs/Device GUIs/GUI_Cameras/GUI_Cameras.exe") -> ()  [unwired: 1 in]
              }
            }
          }
          event "Opt. Spectrometer": Value Change {
            n127 = event-data() -> ("NewVal"=w250:bool)  [unwired: 1 in, 5 out]
            n128 = case shown="True" w250 {
              frame False {
              }
              frame True {
                n129 = call "Run Program.vi"("Program Path"=path "Z:/software/control-all-loasis/HTW/Active Version/builds/Interface builds/Non-General GUIs/BELLA/GUI_HTT_HamamatsuSpec/GUI_HTT_HamamatsuSpec.exe") -> ()  [unwired: 1 in]
              }
            }
          }
          event "RemoteDesktop": Value Change {
            n130 = event-data() -> ("NewVal"=w255:bool)  [unwired: 1 in, 5 out]
            n131 = case shown="True" w255 {
              frame False {
              }
              frame True {
                n132 = call "Run Program.vi"("Program Path"=path "C:/Windows/System32/mstsc.exe") -> ()  [unwired: 1 in]
              }
            }
          }
          event "Google Drive": Value Change {
            n133 = event-data() -> ("NewVal"=w260:bool)  [unwired: 1 in, 5 out]
            n134 = case shown="True" w260 {
              frame False {
              }
              frame True {
                # "HTT daily ops"
                n135 = call-poly <vilib>:"Open URL in Default Browser.vi"("URL"="https://drive.google.com/drive/folders/0B6BJlLNDz1MaOC10bXdFbHFBQ00?usp=sharing") -> ()  [unwired: 5 in, 2 out]
              }
            }
          }
          event "Ethernet Powerstrip": Value Change {
            n136 = event-data() -> ("NewVal"=w265:bool)  [unwired: 1 in, 5 out]
            n137 = case shown="True" w265 {
              frame False {
              }
              frame True {
                # "Ethernet Powerstrip"
                n138 = call-poly <vilib>:"Open URL in Default Browser.vi"("URL"="http://192.168.7.229/outlet.html") -> ()  [unwired: 5 in, 2 out]
              }
            }
          }
          event "HTT Interactive": Value Change {
            n139 = event-data() -> ("NewVal"=w270:bool)  [unwired: 1 in, 5 out]
            n140 = case shown="True" w270 {
              frame False {
              }
              frame True {
                n141 = call-poly <vilib>:"Open URL in Default Browser.vi"("URL"="https://docs.google.com/presentation/d/1vde03GLRziloe-kxBmiBfXX4-hwSL2uU9dDMmq9JgxY/edit?usp=sharing") -> ()  [unwired: 5 in, 2 out]
              }
            }
          }
          event "Search Log": Value Change {
            n142 = event-data() -> ("NewVal"=w275:bool)  [unwired: 1 in, 5 out]
            n143 = case shown="True" w275 {
              frame False {
              }
              frame True {
                n144 = call-poly <vilib>:"Open URL in Default Browser.vi"("URL"="https://docs.google.com/spreadsheets/d/1wR7To7WJHrQNP-2Id8ScCGPPim0LYwsaw_KNOLmAjJY/edit?usp=sharing") -> ()  [unwired: 5 in, 2 out]
              }
            }
          }
          event "Jet enable": Value Change {
            # "For instructions on how to use the JKI State Machine, examples and video tutorials, visit:\nhttp://jkisoft.com/state-machine/\n\nJKI State Machine™\nhttp://jkisoft.com/state-machine/\nCopyright (C) 2005-2008, JKI <info@jkisoft.com>\nALL RIGHTS RESERVED"
            n145 = event-data() -> ("NewVal"=w280:bool)  [unwired: 1 in, 5 out]
            n146 = Bundle By Name(cluster=w282, "Jet enable"=w280) -> (w281:T8)
            n147 = case shown="True" w280 {
              tunnel: [0.0 ("opening Time") 0.002 ("opening Time")] -> w279
              frame False {
              }
              frame True {
              }
            }
            n148 = property on="Width.Ch 5::8" class="DigNum (strict)"("Val(Sgnl)"=w279) -> ()  [unwired: 2 in, 2 out]
          }
          event Panel Close? {
            # "Discard the event because we'll close the front panel ourselves in Macro: Exit"
            # "Close Panel button (pressed) Event\n(this executes Macro: Exit to terminate the VI)"
            n149 = event-data() -> ()  [unwired: 1 in, 1 out]
            n150 = call <vilib>:"Add State(s) to Queue__jki_lib_state_machine.vi"("State(s) in Front (\"\")"="Macro: Exit", "State(s) in (\"\")"=w291) -> ("States Out"=w290:string)  [unwired: 13 in]
            n151 = event-data("Discard?"=TRUE) -> ()  [unwired: 1 in, 1 out]
          }
        }
      }
      frame "SetTogglesJet" {
        n152 = Greater?(x="Width.Ch 5::8", y=0.0001) -> (0:w293:bool)
        n153 = Greater?(x="Amplitude.Ch 5::8", y=2.5) -> (0:w301:bool)
        n154 = Select(t=TRUE, s=w293, f=FALSE) -> (s? t:f=w292:bool)
        n155 = Select(t=TRUE, s=w301, f=FALSE) -> (s? t:f=w298:bool)
        n156 = local write "Jet enable"(w292) -> ()
        n157 = local write "Jet trigger"(w298) -> ()
      }
      frame "---------- Core ----------" {
        # "Do not put any code in this frame.\n(it is a separator no-op)"
        n158 = call <vilib>:"Add State(s) to Queue__jki_lib_state_machine.vi"("State(s) in (\"\")"=w310) -> ("States Out"=w309:string)  [unwired: 14 in]
      }
      frame Default {
        w320 = 42 items=["No error", "Argument error", "Memory is full", "Out of zone", "End of file", "File already open", "Generic file I/O error", "File not found", "File permission error", "Disk is full", "Duplicate path", "Too many files open", "System feature not enabled", "Resource file not found", "Cannot add resource", "Resource not found", "Image not found", "Image memory error", "Pen does not exist", "Config type invalid", "Config token not found", "Config parse error", "Config memory error", "Bad external code format", "Bad external code offset", "External code not present", "Null window", "Destroy window error", "Null menu", "Print aborted", "Bad print record", "Print driver error", "Windows error during printing", "Memory error during printing", "Print dialog error", "Generic print error", "Invalid device refnum", "Device not found", "Device parameter error", "Device unit error", "Cannot open device", "Device call aborted", "Generic error", "Cancelled by user", "Object ID too low", "Object ID too high", "Object not in heap", "Unknown heap", "Unknown object (invalid DefProc)", "Unknown object (DefProc not in table)", "Message out of range", "Invalid (null) method", "Unknown message", "Manager call not supported", "Bad address", "Network operation in progress", "Network operation timed out", "Connection is busy", "Network attribute not supported", "Network error", "Address in use", "System out of memory", "Connection aborted", "Connection refused", "Not connected", "Already connected", "Connection closed", "Initialization error (interapplication manager)", "Bad occurrence", "Wait on unbound occurrence handler", "Occurrence queue overflow", "Datalog type conflict", "Unused", "Unrecognized type (interapplication manager)", "Memory corrupt", "Failed to make temporary DLL", "Old CIN version", "Drag socket not found", "Failed to load drop-object", "Failed to register OLE object", "Failed to release OLE object", "Format specifier type mismatch", "Unknown format specifier", "Too few format specifiers", "Too many format specifiers", "Scan failed", "Newer CIN version", "Error converting to variant", "Runtime menu error", "Password tampered", "Variant attribute not found", "Incompatible variant data type", "Event data is not available", "Event Store is not present", "Occurrence is not found", "Event Queue is not created", "Event info is not available", "Refnum passed is NULL", "Error retrieving Class GUID", "Error retrieving CoClass GUID", "Error retrieving TypeLib GUID.", "Bad built application magic bytes.", "Specific driver is different from the specific driver associated with the Logical Name.", "There is no session opened to the class driver.", "Max Error", "MAX - Error with config objects", "MAX - Error loading configuration", "MAX - Group not supported"]
        # "Current State"
        # "Do not delete, rename, or modify this frame.\n(this is used to capture unhandled states and typos)"
        # "Handle mistyped state name (developer tool)"
        n159 = Format Into String(format string="Software Exception: Unhandled State \"%s\"." ("message"), error in=w316, w311) -> (resulting string=w319:string, error out=w318:errorcluster)  [unwired: 1 in]
        n160 = call <vilib>:"Error Cluster From Error Code.vi"("show call chain? (False)"=TRUE, "error in (no error)"=w318, "error message (\"\")"=w319, "error code (0)"=w320) -> ("error out"=w317:errorcluster)  [unwired: 5 in]
        n161 = call <vilib>:"Add State(s) to Queue__jki_lib_state_machine.vi"("State(s) in (\"\")"=w315) -> ("States Out"=w314:string)  [unwired: 14 in]
      }
      frame "Initialize Core Data" {
        # "Do not delete, rename, or modify this frame.\n(this is used to determine panel behavior on exit)"
        # "originally closed?"
        # "exe?"
        # "If panel starts closed or is an EXE, then close it when we exit"
        n162 = call <vilib>:"Add State(s) to Queue__jki_lib_state_machine.vi"("State(s) in (\"\")"=w333) -> ("States Out"=w332:string)  [unwired: 14 in]
        n163 = property class="App"() -> ("App.Kind"=w328:T6)  [unwired: 2 in, 2 out]
        n164 = Equal?(x=w328, y=T6."Run Time System" ("Application:Kind")) -> (x = y?=w325:bool)
        n165 = property class="VI"() -> ("Front Panel.Open"=w329:bool)  [unwired: 2 in, 2 out]
        n166 = Not(x=w329) -> (.not. x?=w326:bool)
        n167 = control-ref of="Current VI Reference"() -> (w322:refnum<vi>)
        n168 = Or(x=w326, y=w325) -> (x .or. y?=w323:bool)
        n169 = Bundle By Name(cluster=w324, "Core.Current VI Reference"=w322, "Core.Close Panel on Exit?"=w323) -> (w331:T8)
      }
      frame "Error Handler" {
        # "Unhandled Error -- Display it"
        # "Handle any errors here.\nYou can also output any states to clean-up after errors occur"
        # "Clear error"
        n170 = call <vilib>:"General Error Handler.vi"("error in (no error)"=w335) -> ()  [unwired: 10 in, 5 out]
        n171 = call <vilib>:"Add State(s) to Queue__jki_lib_state_machine.vi"("State(s) in Front (\"\")"="/* Post Error States", "State(s) in (\"\")"=w339) -> ("States Out"=w338:string)  [unwired: 13 in]
      }
      frame "Exit" {
        # "Do not put any code in this frame.\n(No errors that occur here will be handled.)"
        n172 = call <vilib>:"Add State(s) to Queue__jki_lib_state_machine.vi"("State(s) in (\"\")"=w344) -> ("States Out"=w343:string)  [unwired: 14 in]
      }
      frame "---------- Data ----------" {
        # "Do not put any code in this frame.\n(It is a separator no-op. You can make a copy of this frame to create a new Data frame)"
        n173 = call <vilib>:"Add State(s) to Queue__jki_lib_state_machine.vi"("State(s) in (\"\")"=w348) -> ("States Out"=w347:string)  [unwired: 14 in]
      }
      frame "Data: Initialize" {
        w349 = FALSE  # Jet enable
        w350 = FALSE  # Fire Continues Allowed
        w352 = u32 0  # Tik1
        w351 = u32 0  # Tik2
        w353 = FALSE  # Jet trigger
        w354 = 0.0  # Discharge timing offset
        w355 = 0.0  # Heater timing offset
        w356 = T11 {"Current VI Reference"=refnum, "Close Panel on Exit?"=FALSE}  # Core
        # "do not delete - used by framework"
        # "Expand Bundle to add new data elements to shift register data."
        # "Add new data here."
        # "Data names and types of shift register data are defined by this bundle."
        # "Initialize the shift-register data, here.\n(data names are defined by what you wire into the bundle function)"
        n174 = call <vilib>:"Add State(s) to Queue__jki_lib_state_machine.vi"("State(s) in (\"\")"=w360) -> ("States Out"=w359:string)  [unwired: 14 in]
        n175 = Bundle("Core"=w356, "Heater timing offset"=w355, "Discharge timing offset"=w354, "Jet trigger"=w353, "Tik1"=w352, "Tik2"=w351, "Fire Continues Allowed"=w350, "Jet enable"=w349) -> (w358:T8)  [unwired: 1 in]
      }
      frame "Data: Cleanup" {
        # "Cleanup any data and references, here.\n(this is called automatically, by the Macro: Exit)"
        n176 = Unbundle By Name(w361) -> ("Core.Current VI Reference"=w364:refnum<vi>)
        n177 = Close Reference(reference=w364, error in (no error)=w363) -> (error out=w362:errorcluster)
        n178 = call <vilib>:"Add State(s) to Queue__jki_lib_state_machine.vi"("State(s) in (\"\")"=w366) -> ("States Out"=w365:string)  [unwired: 14 in]
      }
      frame "---------- UI ----------" {
        # "Do not put any code in this frame.\n(It is a separator no-op. You can make a copy of this frame to create a new UI frame)"
        n179 = call <vilib>:"Add State(s) to Queue__jki_lib_state_machine.vi"("State(s) in (\"\")"=w370) -> ("States Out"=w369:string)  [unwired: 14 in]
      }
      frame "UI: Initialize" {
        # "Initialize the User Interface, here.\n(this is called automatically, by the Macro: Init)"
        n180 = call <vilib>:"Add State(s) to Queue__jki_lib_state_machine.vi"("State(s) in (\"\")"=w374) -> ("States Out"=w373:string)  [unwired: 14 in]
      }
      frame "UI: Cursor Set" {
        # "Argument"
        # "Set and Unset Cursor Busy.\n(Usage: \"UI: Cursor Set >> Busy|Idle\")"
        n181 = case shown="\"Idle\", Default" w375 {
          tunnel: w377 -> [w382 w384]
          tunnel: [w381 w383] -> w376
          frame "Idle", Default {
            n182 = call <vilib>:"Unset Busy.vi"("error in (no error)"=w382) -> ("error out"=w381:errorcluster)  [unwired: 10 in]
          }
          frame "Busy" {
            n183 = call <vilib>:"Set Busy.vi"("error in (no error)"=w384) -> ("error out"=w383:errorcluster)  [unwired: 9 in, 1 out]
          }
        }
        n184 = call <vilib>:"Add State(s) to Queue__jki_lib_state_machine.vi"("State(s) in (\"\")"=w380) -> ("States Out"=w379:string)  [unwired: 14 in]
      }
      frame "UI: Front Panel State" {
        # "Argument"
        # "Set Front Panel Open or Closed\n(Usage: \"UI: Front Panel State >> Open|Close\")"
        n185 = Unbundle By Name(w387) -> ("Core.Current VI Reference"=w386:refnum<vi>)
        n186 = case shown="\"Close\"" w385 {
          tunnel: w389 -> [w395 w408]
          tunnel: [w397 w409] -> w388
          tunnel: w386 -> [w396 w406]
          frame "Open", Default {
            n187 = property class="VI"(reference=w396, error in=w395) -> (reference out=w393:refnum<vi>, error out=w394:errorcluster, "Front Panel.Open"=w392:bool)
            n188 = case shown="False" w392 {
              tunnel: [w400 w403] -> w397
              tunnel: w394 -> [w399 w403]
              tunnel: w393 -> [w398 _]
              frame False {
                n189 = invoke class="VI" method="FP.Open"(reference=w398, error in=w399, "Activate"=TRUE, "State"=T7."Standard") -> (error out=w400:errorcluster)  [unwired: 1 in, 4 out]
              }
              frame True {
              }
            }
          }
          frame "Close" {
            n190 = property class="VI"(reference=w406, error in=w408) -> (reference out=w405:refnum<vi>, error out=w407:errorcluster, "Front Panel.Open"=w404:bool)
            n191 = case shown="True" w404 {
              tunnel: [w410 w413] -> w409
              tunnel: w407 -> [w410 w412]
              tunnel: w405 -> [_ w411]
              frame False {
              }
              frame True {
                n192 = invoke class="VI" method="FP.Close"(reference=w411, error in=w412) -> (error out=w413:errorcluster)  [unwired: 1 in, 2 out]
              }
            }
          }
        }
        n193 = call <vilib>:"Add State(s) to Queue__jki_lib_state_machine.vi"("State(s) in (\"\")"=w391) -> ("States Out"=w390:string)  [unwired: 14 in]
      }
      frame "---------- Macro ----------" {
        # "Do not put any code in this frame.\n(It is a separator no-op. You can make a copy of this frame to create a new Macro frame)"
        n194 = call <vilib>:"Add State(s) to Queue__jki_lib_state_machine.vi"("State(s) in (\"\")"=w417) -> ("States Out"=w416:string)  [unwired: 14 in]
      }
      frame "Macro: Initialize" {
        w418 = "Data: Initialize\nInitialize Core Data\nUI: Initialize\nUI: Front Panel State >> Open"  # Data: Initialize Initialize Core Data UI: Initialize UI: Front Panel State >> Open
        # "Initialization Macro\n(This is called once, when the VI starts)"
        n195 = call <vilib>:"Add State(s) to Queue__jki_lib_state_machine.vi"("State(s) in Front (\"\")"=w418, "State(s) in (\"\")"=w422) -> ("States Out"=w421:string)  [unwired: 13 in]
      }
      frame "Macro: Exit" {
        # "Exit Macro\n(This is called once, when the VI exits)"
        n196 = Unbundle By Name(w429) -> ("Core.Close Panel on Exit?"=w428:bool)
        n197 = Select(t="UI: Front Panel State >> Close", s=w428, f="") -> (s? t:f=w425:string)
        n198 = call <vilib>:"Add State(s) to Queue__jki_lib_state_machine.vi"("State(s) in (\"\")"=w425, "State(s) at Back (\"\")"="Data: Cleanup\nExit") -> ("States Out"=w423:string)  [unwired: 13 in]
        n199 = call <vilib>:"Add State(s) to Queue__jki_lib_state_machine.vi"("State(s) in Front (\"\")"=w423, "State(s) in (\"\")"=w432) -> ("States Out"=w431:string)  [unwired: 13 in]
      }
      frame "---------- New Category ----------" {
        # "Template Separator\n(You can make a copy of, or modify, this frame)"
        n200 = call <vilib>:"Add State(s) to Queue__jki_lib_state_machine.vi"("State(s) in (\"\")"=w436) -> ("States Out"=w435:string)  [unwired: 14 in]
      }
      frame "Action: Fire" {
        # "Your code here.\n(You can make a copy of, or modify, this frame)"
        n201 = property on="fire::10" class="Str"(error in=w438, "Val(Sgnl)"="fire>>force" ("Value (Signaling)")) -> (error out=w437:errorcluster)  [unwired: 1 in, 1 out]
        n202 = call <vilib>:"Add State(s) to Queue__jki_lib_state_machine.vi"("State(s) in (\"\")"=w442) -> ("States Out"=w441:string)  [unwired: 14 in]
      }
    }
  }
